vi "SceneRoot_Init.vi"(8 "error in (no error)":errorcluster, 10 "display in":refnum<vi>, 11 "class data in":refnum<class "SceneRoot.lvclass">) -> (0 "error out":errorcluster, 3 "class data out":refnum<class "SceneRoot.lvclass">)   [LabVIEW 2010, in "RenderBase.lvlib" / "SceneRoot.lvclass"]
doc: "Initializes the scene root."
uses:
  SceneRoot.lvclass
  SceneRoot.lvclass/SceneRoot.ctl
  <vilib>/picture/3D Picture Control/NI_3D Picture Control.lvlib
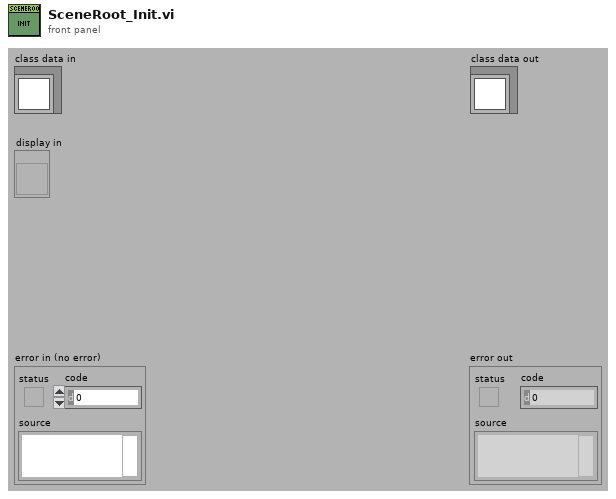
[diagram p1: front panel]
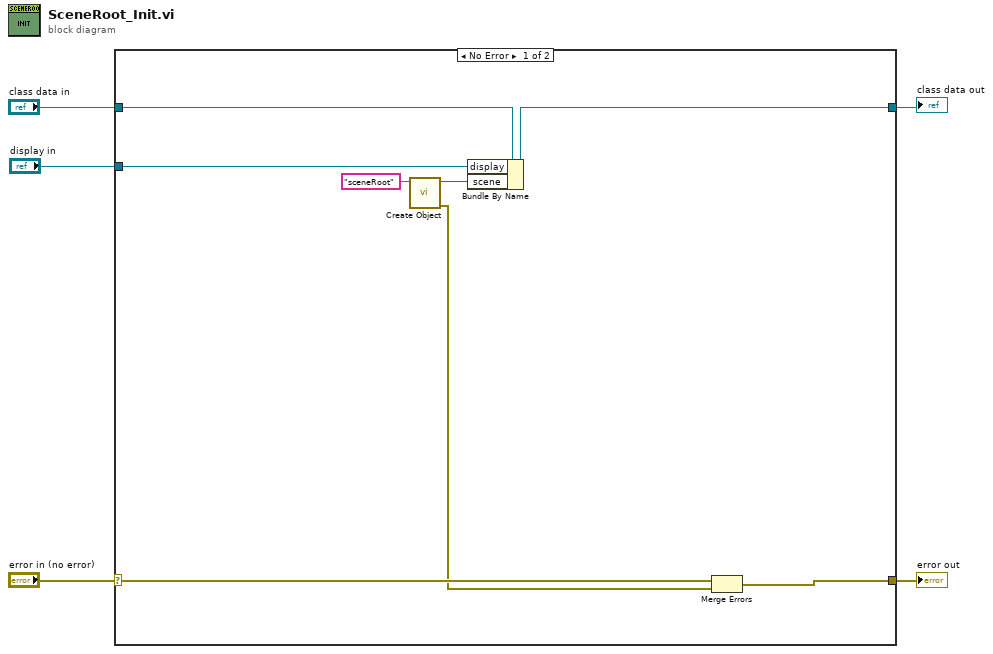
[diagram p0: block diagram]
diagram:
  n1 = case shown="No Error" "error in (no error)" {
    selector: "error in (no error)" -> [w13 w15]
    tunnel: [w7 w15] -> w4
    tunnel: "class data in" -> [w12 w14]
    tunnel: [w11 w14] -> w2
    tunnel: "display in" -> [w10 _]
    frame No Error {
      n2 = call <vilib>:"Create Object.vi"("Name"="sceneRoot") -> ("error out"=w6:errorcluster, "Scene:New Object"=w8:refnum<vi>)  [unwired: 9 in]
      n3 = Bundle By Name(cluster=w12, "display"=w10, "scene"=w8) -> (w11:refnum<class "SceneRoot.lvclass">)
      n4 = Merge Errors(w13, w6) -> (w7:errorcluster)
    }
    frame Error {
    }
  }
  "error out" <- w4
  "class data out" <- w2
